vi "Globals.vi"() -> ()   [LabVIEW 2016]
panel:
  out "EmerStop":bool
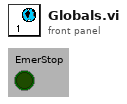
[diagram p1: front panel]
diagram:
